vi "Extended Register Read Long.vi"(0 "instrument handle in":refnum<k15>, 1 "Bus Number":i32, 5 "Slave Address":T3=12 format="%02x", 7 "Register Address":T2 format="%02x", 9 "Byte Count":i32=1, 11 "error in (no error)":errorcluster) -> (4 "instrument handle out":refnum<k15>, 6 "Register Data":T1[](array[typedef]) format="%02x", 8 "Parity":bool, 15 "error out":errorcluster)   [LabVIEW 2018, in "MIPI RFFE API.lvlib"]
uses:
  MIPI RFFE API.lvlib
  Slave Address.ctl
  Register Address.ctl
  Register Data.ctl
  Extended Command/RFFE Extended Command.lvclass/RFFE Extended Command.ctl
  RegReadExt/RFFE RegReadExt Command.lvclass/RFFE RegReadExt Command.ctl
  Extended Command/Get Register Data.vi
  RegReadExt/Get Parity.vi
  RegReadExtLong/RFFE RegReadExtLong Command.lvclass
  C:/Users/semoore/Projects/mipi-rffe-labview-oop/Extended Command/RFFE Extended Command.lvclass
  C:/Users/semoore/Projects/mipi-rffe-labview-oop/RegReadExt/RFFE RegReadExt Command.lvclass
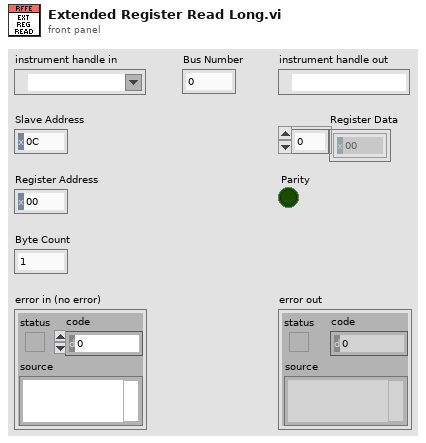
[diagram p1: front panel]
types:
  T1 = typedef "MIPI RFFE API.lvlib/Register Data.ctl" = u8
  T2 = typedef "MIPI RFFE API.lvlib/Register Address.ctl" = u16
  T3 = typedef "MIPI RFFE API.lvlib/Slave Address.ctl" = u8
  T4 = typedef "RFFE Commands.lvlib/Register Data.ctl" = u8
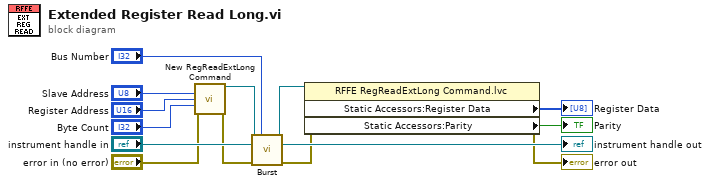
[diagram p0: block diagram]
diagram:
  n1 = call "New RegReadExtLong Command.vi"("Slave Address"="Slave Address", "Register Address"="Register Address", "Byte Count"="Byte Count", "error in (no error)"="error in (no error)") -> ("RFFE RegReadExtLong Command out"=w4:refnum<class "RFFE RegReadExtLong Command.lvclass">, "error out"=w5:errorcluster)  [unwired: 10 in]
  n2 = call-dynamic "Burst.vi"("RFFE RegReadExt Command in"=w4, "Bus Number"="Bus Number", "instrument handle in"="instrument handle in", "error in (no error)"=w5) -> ("RFFE RegReadExt Command out"=w3:refnum<class "RFFE RegReadExtLong Command.lvclass">, "instrument handle out"=→"instrument handle out":refnum<k15>, "error out"=w2:errorcluster)  [unwired: 9 in]
  n3 = property class="RFFE RegReadExtLong Command.lvc"(reference=w3, error in=w2) -> (error out=→"error out":errorcluster, "Static Accessors:Register Data"=→"Register Data":T4[], "Static Accessors:Parity"=→"Parity":bool)  [unwired: 1 out]
